vi "Register.vi"(11 "API in":refnum<class "API.lvclass">) -> (3 "Message":refnum<event-registration>)   [LabVIEW 2024, in "API.lvclass"]
uses:
  API.lvclass
  API.lvclass/API.ctl
  Message.ctl
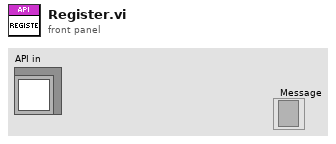
[diagram p1: front panel]
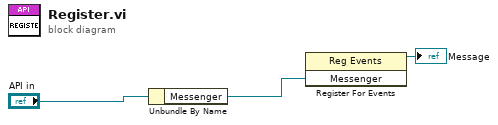
[diagram p0: block diagram]
diagram:
  n1 = Unbundle By Name("API in") -> ("Messenger"=w2:refnum<user-event>)
  n2 = register-events(w2) -> (reference out=→"Message":refnum<event-registration>)  [unwired: 2 in, 1 out]
